vi "LS335 Create channel list.vi"(11 "Data":T1={"Heater"=FALSE, "A"=FALSE, "B"=FALSE, " RAW"=FALSE, "Set point"=0.0, "Set Heater Range"=enum."0 (Off)", "Approach"=enum."Instant", "Ramp rate, K/min"=1.0}) -> (3 "Array":string[](array[string]))   [LabVIEW 2015]
uses:
  LakeShore335 Front Panel Data.ctl
  LakeShore335 Heater Ranges.ctl
  Neocera/Neocera Set Point Aproach.ctl
panel:
  # "Temperature Monitor"
  # "Record Channels"
  # "Temperature Control"
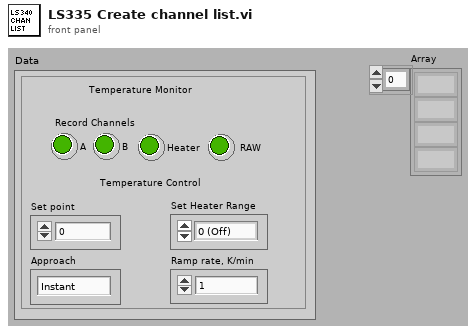
[diagram p1: front panel]
types:
  T1 = typedef "LakeShore335 Front Panel Data.ctl" = cluster{"Heater":bool, "A":bool, "B":bool, " RAW":bool, "Set point":dbl, "Set Heater Range":T2, "Approach":T3, "Ramp rate, K/min":dbl}
  T2 = typedef "LakeShore335 Heater Ranges.ctl" = enum16{"0 (Off)", "1 Low", "2 Medium", "3 High"}
  T3 = typedef "Neocera Set Point Aproach.ctl" = enum16{"Instant", "Ramp"}
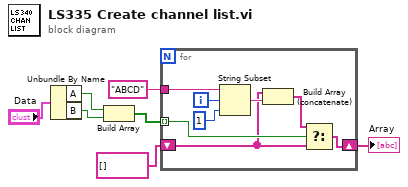
[diagram p0: block diagram]
diagram:
  n1 = Unbundle By Name("Data") -> ("A"=w6:bool, "B"=w5:bool)
  n2 = Build Array(w6, w5) -> (w3:bool[])
  n3 = for {
    tunnel: "ABCD" -> [w15]
    tunnel: w3 -> [w11] mode=indexing
    shift-right: [w8] -> w1
    shift-left: string[] [] -> [w9]
    i -> [w14]
    n4 = String Subset(string=w15, offset (0)=w14, length (rest)=1 ("length (rest)")) -> (substring=w13:string)
    n5 = Build Array (concatenate)(w9, w13) -> (w10:string[])
    n6 = Select(t=w10, s=w11, f=w9) -> (s? t:f=w8:string[])
  }
  "Array" <- w1
